vi "testing_string_to_enum.vi"() -> ()   [LabVIEW 2019, in "mmW_commands.lvlib"]
uses:
  TypeDefs/commands.ctl
  mmW_commands.lvlib
panel:
  out "String":string="mmW_instrument_commands 2"
  in  "mmW_instrument_commands 2":T1=enum."configure_rf"
  out "mmW_instrument_commands":T1=enum."configure_rf"
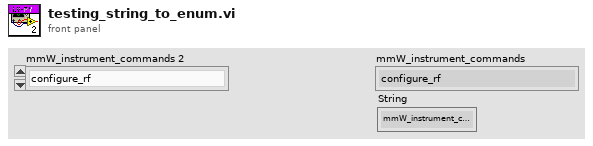
[diagram p1: front panel]
types:
  T1 = typedef "mmW_commands.lvlib/commands.ctl" = enum16{"configure_fs", "configure_rf", "configure_trigger", "equalization_enable", "equalization_start", "lo_sync_enable", "equalization_stop", "get_instrument_status", "get_versions", "initialize_hw", "pop_rx", "set_log_level", "Shutdown", "start", "start_instrument_app", "stop", "transceive", "trigger_burst", "trigger_sync_enable", "Write TX", "resp_generic", "resp_waveform"}
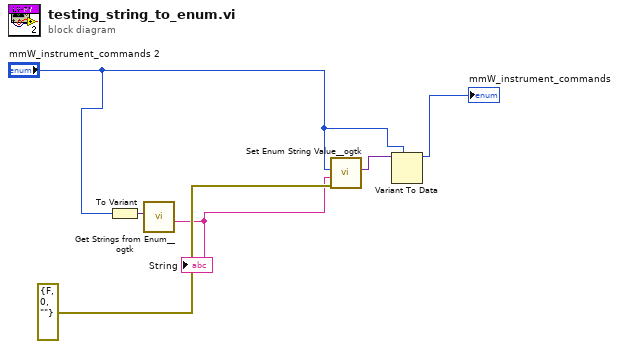
[diagram p0: block diagram]
diagram:
  n1 = To Variant(anything="mmW_instrument_commands 2") -> (Variant=w4:variant)
  n2 = call <userlib>:"Get Strings from Enum__ogtk.vi"("Enum"=w4) -> ("String Value"=w1:string)  [unwired: 7 in, 3 out]
  "String" <- w1
  n3 = call <userlib>:"Set Enum String Value__ogtk.vi"("error in (no error)"=errorcluster {"status"=FALSE, "code"=0, "source"=""}, "String Value"=w1, "Default Enum Value"="mmW_instrument_commands 2") -> ("Enum"=w6:variant)  [unwired: 7 in, 1 out]
  n4 = Variant To Data(type="mmW_instrument_commands 2", Variant=w6) -> (data=→"mmW_instrument_commands":T1)  [unwired: 1 in, 1 out]
